vi "new.vi"(8 "Error In":errorcluster, 10 "ref":refnum<vi>, 11 "Wire in":refnum<class "Wire.lvclass">) -> (0 "Error Out":errorcluster, 3 "Wire Out":refnum<class "Wire.lvclass">)   [LabVIEW 2023, in "TLC_Scripto.lvlib" / "Wire.lvclass"]
uses:
  Wire.lvclass
  Wire.lvclass/Wire.ctl
  GObject/GObject.lvclass
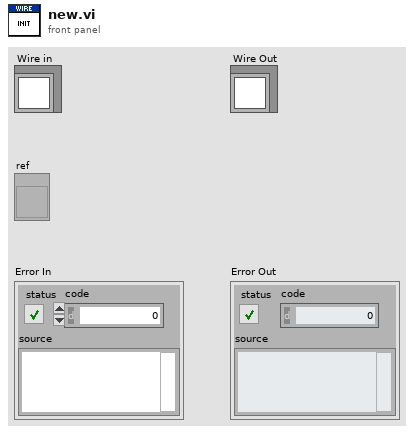
[diagram p1: front panel]
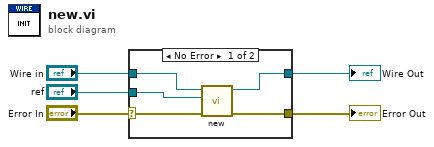
[diagram p0: block diagram]
diagram:
  n1 = case shown="No Error" "Error In" {
    selector: "Error In" -> [w10 w12]
    tunnel: [w8 w11] -> w5
    tunnel: [w9 w12] -> w3
    tunnel: "ref" -> [w6 _]
    tunnel: "Wire in" -> [w7 w11]
    frame No Error {
      n2 = call-parent "new.vi"("Error In"=w10, "ref"=w6, "GObject in"=w7) -> ("Error Out"=w9:errorcluster, "GObject out"=w8:refnum<class "Wire.lvclass">)  [unwired: 7 in]
    }
    frame Error {
    }
  }
  "Wire Out" <- w5
  "Error Out" <- w3
